vi "Mouse Move Hanlde.vi"(8 "error in (no error)":errorcluster, 11 "UI_Top_Customer in":refnum<class "UI_Top_Customer.lvclass">) -> (0 "error out":errorcluster, 3 "UI_Top_Customer out":refnum<class "UI_Top_Customer.lvclass">)   [LabVIEW 2021, in "UI_Top_Customer.lvclass"]
uses:
  UI_Top_Customer.lvclass
  UI_Top_Customer.lvclass/UI_Top_Customer.ctl
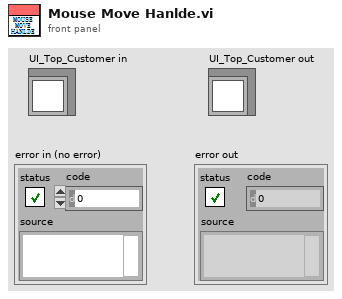
[diagram p1: front panel]
types:
  T1 = enum32{"Invalid", "Standard", "Closed", "Hidden", "Minimized", "Maximized"}
  T2 = typedef "UI_Top_Customer.lvclass/Pane MouseDown.ctl" = cluster{"Type":T3, "Coords":cluster{"Horizontal":i32, "Vertical":i32}, "Mods":cluster{"Double Click":bool, "Menu Key":bool}, "Pane: MouseDown":bool}
  T3 = typedef "lveventtype.ctl" = enum32{"Null", "Timeout", "Annotation Menu Selection", "Annotation Menu Selection?", "App Instance Close", "App Instance Close?", "Autoscale Range Change", "Bookmark Info Change", "Cell Edit", "Cell Edit?", "Cursor Grab", "Cursor Grab?", "Cursor Menu Selection", "Cursor Menu Selection?", "Cursor Move", "Cursor Release", "Data Change", "Direction Change", "Display State Change", "Drag Ended", "Drag Enter", "Drag Leave", "Drag Over", "Drag Source Update", "Drag Starting", "Drag Starting?", "Drop", "Exec State Change", "Key Down", "Key Down?", "Key Repeat", "Key Repeat?", "Key Up", "Listbox Double Click", "Menu Activation?", "Menu Selection (App)", "Menu Selection? (App)", "Menu Selection (User)", "Mouse Down", "Mouse Down?", "Mouse Enter", "Mouse Leave", "Mouse Move", "Mouse Up", "Mouse Wheel", "NI Security User Change (App)", "Pane Size", "Panel Close", "Panel Close?", "Panel Resize", "Plot Attribute Change", "Scale Range Change", "Shortcut Menu Activation?", "Shortcut Menu Selection (App)", "Shortcut Menu Selection? (App)", "Shortcut Menu Selection (User)", "Tree Double Click", "Tree Drag", "Tree Drag?", "Tree Drop", "Tree Drop?", "Tree Item Close", "Tree Item Close?", "Tree Item Open", "Tree Item Open?", "User Event", "Value Change"}
  T4 = cluster{"Horizontal":i32, "Vertical":i32, "Scrolling":i32}
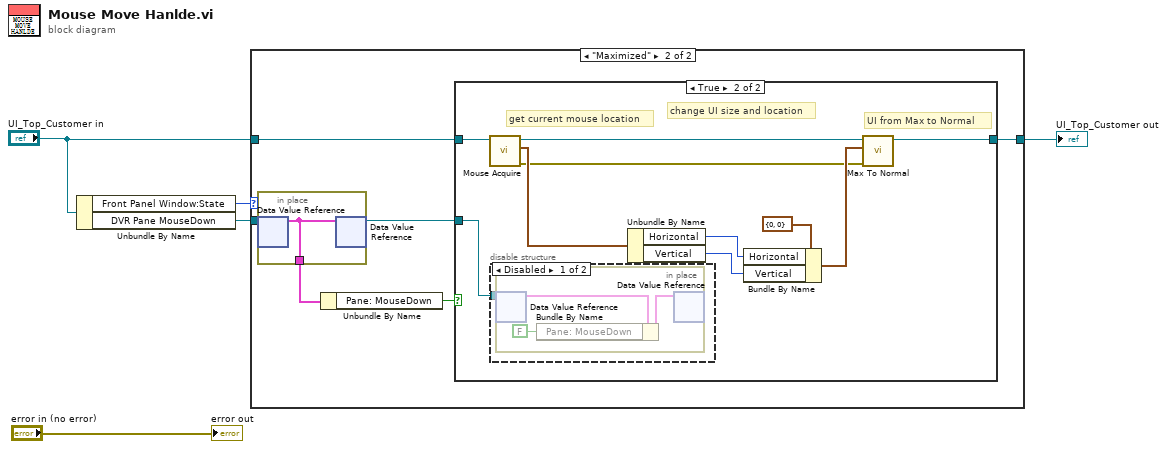
[diagram p0: block diagram]
diagram:
  n1 = Unbundle By Name("UI_Top_Customer in") -> ("Front Panel Window:State"=w1:T1, "DVR Pane MouseDown"=w4:refnum<data-value>)
  n2 = case shown="\"Maximized\"" w1 {
    tunnel: w4 -> [_ w12]
    tunnel: "UI_Top_Customer in" -> [w6 w9]
    tunnel: [w6 w8] -> w2
    frame "Invalid", Default {
    }
    frame "Maximized" {
      n3 = in-place {
        in-place-border: [w28] -> w11
        n4 = in-place-dvr #1(w12) -> (w28:T2)  [unwired: 1 out]
        n5 = in-place-dvr #1(w28) -> (w7:refnum<data-value>)  [unwired: 1 out]
      }
      n6 = Unbundle By Name(w11) -> ("Pane: MouseDown"=w10:bool)
      n7 = case shown="True" w10 {
        tunnel: w9 -> [w13 w23]
        tunnel: [w13 w14] -> w8
        tunnel: w7 -> [_ w22]
        frame False {
        }
        frame True {
          # "UI from Max to Normal"
          # "get current mouse location"
          # "change UI size and location"
          n8 = call "Mouse Acquire.vi"("UI_Top_Customer in"=w23) -> ("error out"=w15:errorcluster, "axis info"=w16:T4, "UI_Top_Customer out"=w21:refnum<class "UI_Top_Customer.lvclass">)  [unwired: 7 in, 1 out]
          n9 = disable-structure shown="Disabled" {
            disable-tunnel: w22 -> [w24 _]
            frame Disabled {
              n10 = in-place {
                n11 = in-place-dvr #2(w24) -> (w27:T2)  [unwired: 1 out]
                n12 = Bundle By Name(cluster=w27, "Pane: MouseDown"=FALSE) -> (w26:T2)
                n13 = in-place-dvr #2(w26) -> ()  [unwired: 2 out]
              }
            }
            frame Enabled {
            }
          }
          n14 = Unbundle By Name(w16) -> ("Horizontal"=w18:i32, "Vertical"=w17:i32)
          n15 = Bundle By Name(cluster=cluster{"Horizontal":i32, "Vertical":i32} {"Horizontal"=0, "Vertical"=0} ("MouseCoords"), "Horizontal"=w18, "Vertical"=w17) -> (w19:cluster{"Horizontal":i32, "Vertical":i32})
          n16 = call "Max To Normal.vi"("error in (no error)"=w15, "MouseCoords"=w19, "MainUI in"=w21) -> ("MainUI out"=w14:refnum<class "UI_Top_Customer.lvclass">)  [unwired: 7 in, 1 out]
        }
      }
    }
  }
  "UI_Top_Customer out" <- w2
  "error out" <- "error in (no error)"
